vi "0037-0006_HTU21D.vi"() -> ()   [LabVIEW 2014]
panel:
  out "x = y?":bool
  out "humi":dbl format="%#.2g"
  out "temp":dbl format="%#.2g"
  out "error out":errorcluster caption="エラー出力"
  in  "停止ボタン":bool
  # "℃"
  # "％RH"
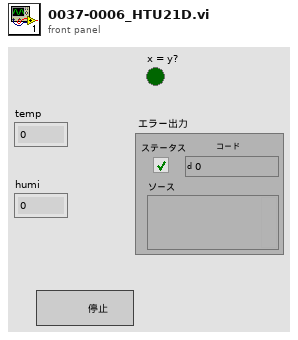
[diagram p1: front panel]
types:
  T1 = cluster{"bitRate":u32, "address":u8, "autoReadRespond":bool, "writeTimeout":u16, "readTimeout":u16, "sclLowTimeout":bool, "transferRetries":u16}
  T2 = typedef "CP2112_device.ctl" = i32
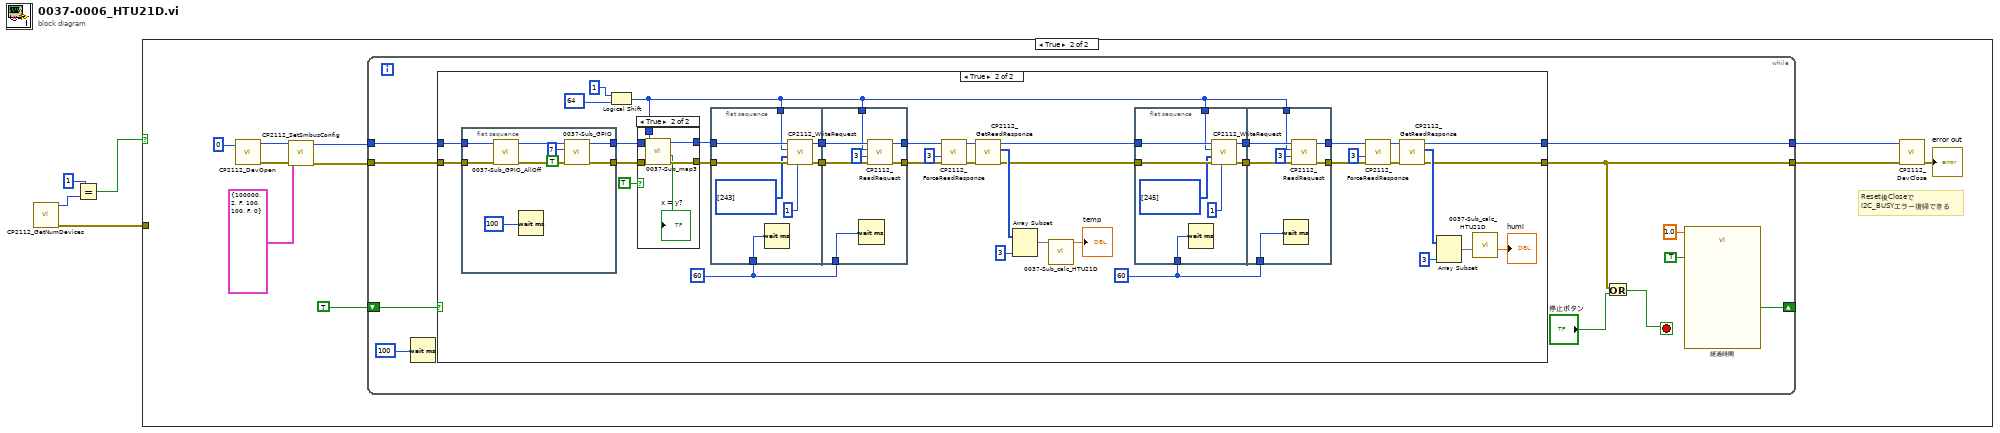
[diagram p0: block diagram]
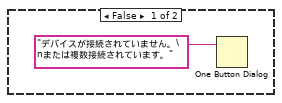
[diagram p2: hidden frame]
diagram:
  n1 = call "CP2112_GetNumDevices.vi"() -> ("error out"=w1:errorcluster, "numDevices"=w3:i32)  [unwired: 9 in, 1 out]
  n2 = Equal?(x=1, y=w3) -> (x = y?=w2:bool)
  n3 = case shown="TRUE" w2 {
    tunnel: w1 -> [_ _]
    frame False {
      n4 = One Button Dialog(message="デバイスが接続されていません。\nまたは複数接続されています。" ("メッセージ")) -> ()  [unwired: 1 in, 1 out]
    }
    frame True {
      # "Reset後Closeで\nI2C_BUSYエラー復帰できる"
      n5 = call "CP2112_DevOpen.vi"("deviceNum"=0) -> ("error out"=w10:errorcluster, "device"=w11:T2)  [unwired: 8 in, 1 out]
      n6 = call "CP2112_SetSmbusConfig.vi"("error in (no error)"=w10, "smbusInfo"=T1 {"bitRate"=100000, "address"=2, "autoReadRespond"=FALSE, "writeTimeout"=100, "readTimeout"=100, "sclLowTimeout"=FALSE, "transferRetries"=0}, "device"=w11) -> ("error out"=w12:errorcluster, "deviceOut"=w13:T2)  [unwired: 6 in, 1 out]
      n7 = while {
        tunnel: w12 -> [w26]
        tunnel: w13 -> [w25]
        tunnel: [w22] -> w8
        tunnel: [w21] -> w7
        shift-right: [w18] -> _
        shift-left: TRUE ("Auto Reset") -> [w19]
        stop <- w23 stop-if-true
        n8 = Wait (ms)(milliseconds to wait=u32 100 ("ミリ秒待機時間")) -> ()  [unwired: 1 out]
        n9 = case shown="TRUE" w19 {
          tunnel: w26 -> [w27 w55]
          tunnel: w25 -> [w28 w56]
          tunnel: [w27 w37] -> w22
          tunnel: [w28 w38] -> w21
          frame False {
          }
          frame True {
            w41 = u32 60 ("ミリ秒待機時間")
            w57 = u32 60 ("ミリ秒待機時間")
            n10 = flat-sequence {
              tunnel: w56 -> [w98]
              tunnel: w55 -> [w95]
              tunnel: [w96] -> w33
              tunnel: [w93] -> w34
              frame #0 {
                n11 = call "0037-Sub_GPIO_AllOff.vi"("エラー出力 2"=w95, "device"=w98) -> ("エラー出力"=w94:errorcluster, "deviceOut"=w97:T2)  [unwired: 8 in]
                n12 = Wait (ms)(milliseconds to wait=u32 100 ("ミリ秒待機時間")) -> ()  [unwired: 1 out]
                n13 = call "0037-Sub_GPIO.vi"("エラー出力 2"=w94, "ブール"=TRUE, "GPIO"=u8 7, "device"=w97) -> ("エラー出力"=w93:errorcluster, "deviceOut"=w96:T2)  [unwired: 6 in]
              }
            }
            n14 = Logical Shift(y=1, x=64) -> (x << y=w30:i32)
            n15 = case shown="TRUE" TRUE {
              tunnel: w34 -> [w67 w74]
              tunnel: w33 -> [w68 w73]
              tunnel: [w68 w72] -> w32
              tunnel: [w67 w71] -> w31
              tunnel: w30 -> [_ w69]
              frame False {
              }
              frame True {
                n16 = call "0037-Sub_map3.vi"("error out"=w74, "アドレス"=w69, "device"=w73) -> ("error out 2"=w71:errorcluster, "x = y?"=→"x = y?":bool, "device 2"=w72:T2)  [unwired: 5 in]
              }
            }
            n17 = flat-sequence {
              tunnel: w31 -> [w106]
              tunnel: w32 -> [w105]
              tunnel: w30 -> [w100]
              tunnel: [w104] -> w61
              tunnel: [w103] -> w60
              tunnel: w57 -> [w99]
              tunnel: w61 -> [w111]
              tunnel: w60 -> [w110]
              tunnel: [w112] -> w59
              tunnel: [w109] -> w58
              tunnel: w30 -> [w108]
              tunnel: w57 -> [w107]
              frame #0 {
                n18 = Wait (ms)(milliseconds to wait=w99) -> ()  [unwired: 1 out]
                n19 = call "CP2112_WriteRequest.vi"("numBytesToWrite"=i16 1 ("numByteToRead"), "error in (no error)"=w106, "buffer"=u8[] [243], "slaveAddress"=w100, "device"=w105) -> ("error out"=w104:errorcluster, "deviceOut"=w103:T2)  [unwired: 4 in, 1 out]
              }
              frame #1 {
                n20 = Wait (ms)(milliseconds to wait=w107) -> ()  [unwired: 1 out]
                n21 = call "CP2112_ReadRequest.vi"("error in (no error)"=w111, "numByteToRead"=i16 3, "slaveAddress"=w108, "device"=w110) -> ("error out"=w112:errorcluster, "deviceOut"=w109:T2)  [unwired: 5 in, 1 out]
              }
            }
            n22 = call "CP2112_ForceReadResponse.vi"("error in (no error)"=w59, "numByteToRead"=i16 3, "device"=w58) -> ("error out"=w66:errorcluster, "deviceOut"=w65:T2)  [unwired: 6 in, 1 out]
            n23 = call "CP2112_GetReadResponse.vi"("error in (no error)"=w66, "device"=w65) -> ("error out"=w39:errorcluster, "buffer"=w63:u8[], "deviceOut"=w40:T2)  [unwired: 4 in, 3 out]
            n24 = Array Subset(array=w63, length=3 ("長さ")) -> (w52:u8[])  [unwired: 1 in]
            n25 = call "0037-Sub_calc_HTU21D.vi"("temp"=w52) -> ("temp"=→"temp":dbl)  [unwired: 8 in, 1 out]
            n26 = flat-sequence {
              tunnel: w39 -> [w82]
              tunnel: w40 -> [w81]
              tunnel: w30 -> [w76]
              tunnel: [w80] -> w50
              tunnel: [w79] -> w49
              tunnel: w41 -> [w75]
              tunnel: w50 -> [w87]
              tunnel: w49 -> [w86]
              tunnel: [w88] -> w43
              tunnel: [w85] -> w42
              tunnel: w30 -> [w84]
              tunnel: w41 -> [w83]
              frame #0 {
                n27 = Wait (ms)(milliseconds to wait=w75) -> ()  [unwired: 1 out]
                n28 = call "CP2112_WriteRequest.vi"("numBytesToWrite"=i16 1 ("numByteToRead"), "error in (no error)"=w82, "buffer"=u8[] [245], "slaveAddress"=w76, "device"=w81) -> ("error out"=w80:errorcluster, "deviceOut"=w79:T2)  [unwired: 4 in, 1 out]
              }
              frame #1 {
                n29 = Wait (ms)(milliseconds to wait=w83) -> ()  [unwired: 1 out]
                n30 = call "CP2112_ReadRequest.vi"("error in (no error)"=w87, "numByteToRead"=i16 3, "slaveAddress"=w84, "device"=w86) -> ("error out"=w88:errorcluster, "deviceOut"=w85:T2)  [unwired: 5 in, 1 out]
              }
            }
            n31 = call "CP2112_ForceReadResponse.vi"("error in (no error)"=w43, "numByteToRead"=i16 3, "device"=w42) -> ("error out"=w48:errorcluster, "deviceOut"=w47:T2)  [unwired: 6 in, 1 out]
            n32 = call "CP2112_GetReadResponse.vi"("error in (no error)"=w48, "device"=w47) -> ("error out"=w37:errorcluster, "buffer"=w45:u8[], "deviceOut"=w38:T2)  [unwired: 4 in, 3 out]
            n33 = Array Subset(array=w45, length=3 ("長さ")) -> (w36:u8[])  [unwired: 1 in]
            n34 = call "0037-Sub_calc_HTU21D.vi"("humi"=w36) -> ("humi"=→"humi":dbl)  [unwired: 8 in, 1 out]
          }
        }
        n35 = Or(x=w22, y="停止ボタン") -> (x .or. y?=w23:bool)
        n36 = call "経過時間"("Time Target (s)"=1.0, "Auto Reset"=TRUE) -> ("Time has Elapsed"=w18:bool)  [unwired: 10 in, 7 out]
      }
      n37 = call "CP2112_DevClose.vi"("error in (no error)"=w8, "device"=w7) -> ("error out"=→"error out":errorcluster)  [unwired: 9 in]
    }
  }
